vi "compile_options.vi"(8 "error in (no error)":errorcluster, 11 "Wash Options":T2) -> (0 "error out":errorcluster, 3 "Options Array":T1[](array[typedef]))   [LabVIEW 2021]
doc: "compile wash options into array"
uses:
  Controls/Wash Options.ctl
  Controls/states.ctl
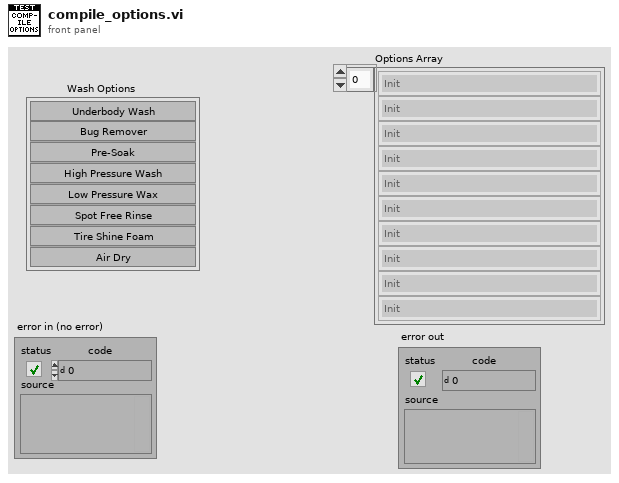
[diagram p1: front panel]
types:
  T1 = typedef "states.ctl" = enum16{"Init", "Select Wash Options", "Configure Options", "Under Body Wash", "Bug Remover", "Pre-Soak", "High Pressure Wash", "Low Pressure Wax", "Spot Free Rinse", "Tire Shine Foam", "Air Dry", "Skip", "Exit", "Stop"}
  T2 = typedef "Wash Options.ctl" = cluster{"Underbody Wash":bool, "Bug Remover":bool, "Pre-Soak":bool, "High Pressure Wash":bool, "Low Pressure Wax":bool, "Spot Free Rinse":bool, "Tire Shine Foam":bool, "Air Dry":bool}
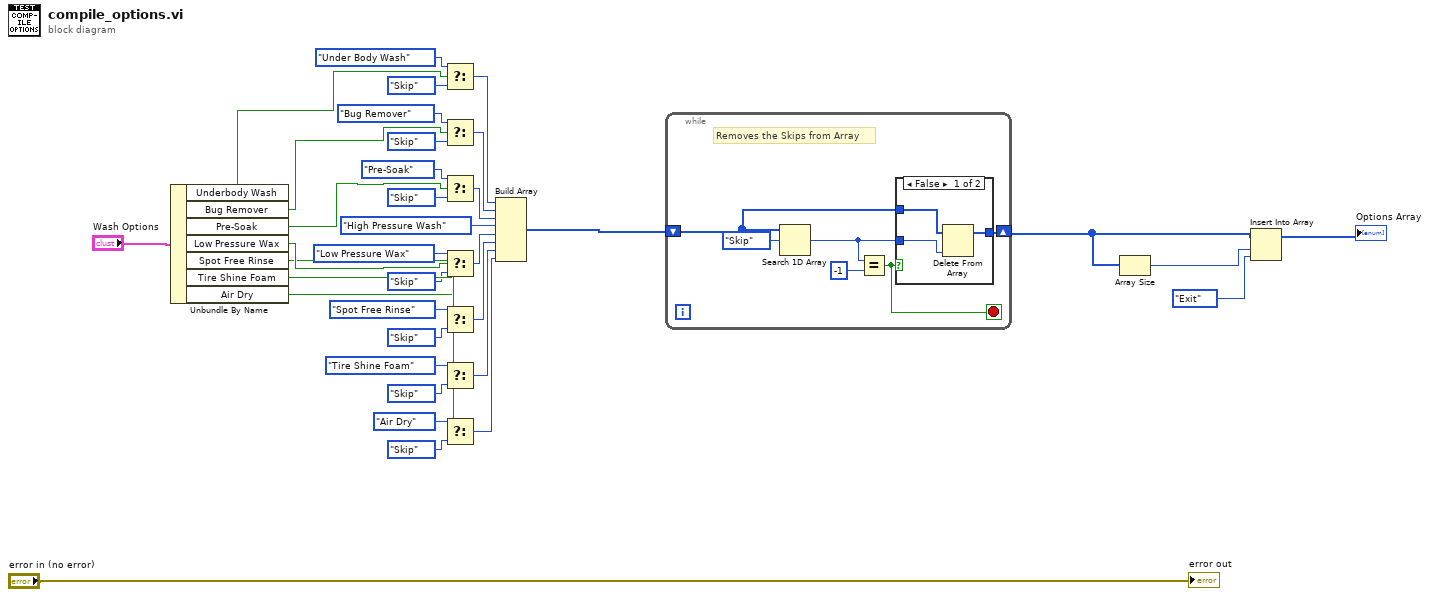
[diagram p0: block diagram]
diagram:
  n1 = Unbundle By Name("Wash Options") -> ("Underbody Wash"=w34:bool, "Bug Remover"=w27:bool, "Pre-Soak"=w26:bool, "Low Pressure Wax"=w25:bool, "Spot Free Rinse"=w24:bool, "Tire Shine Foam"=w23:bool, "Air Dry"=w22:bool)
  n2 = Select(t=states."Under Body Wash" ("Enum"), s=w34, f=states."Skip" ("Enum")) -> (s? t:f=w21:T1)
  n3 = Select(t=states."Bug Remover" ("Enum"), s=w27, f=states."Skip" ("Enum")) -> (s? t:f=w20:T1)
  n4 = Select(t=states."Pre-Soak" ("Enum"), s=w26, f=states."Skip" ("Enum")) -> (s? t:f=w19:T1)
  n5 = Select(t=states."Low Pressure Wax" ("Enum"), s=w25, f=states."Skip" ("Enum")) -> (s? t:f=w17:T1)
  n6 = Select(t=states."Spot Free Rinse" ("Enum"), s=w24, f=states."Skip" ("Enum")) -> (s? t:f=w16:T1)
  n7 = Select(t=states."Tire Shine Foam" ("Enum"), s=w23, f=states."Skip" ("Enum")) -> (s? t:f=w15:T1)
  n8 = Select(t=states."Air Dry" ("Enum"), s=w22, f=states."Skip" ("Enum")) -> (s? t:f=w14:T1)
  n9 = Build Array(w21, w20, w19, states."High Pressure Wash" ("Enum"), w17, w16, w15, w14) -> (w5:T1[])
  n10 = while {
    shift-right: [w38] -> w3
    shift-left: w5 -> [w41]
    stop <- w37 stop-if-true
    # "Removes the Skips from Array"
    n11 = Search 1D Array(1D array=w41, element=states."Skip") -> (index of element=w39:i32)  [unwired: 1 in]
    n12 = Equal?(x=w39, y=-1) -> (x = y?=w37:bool)
    n13 = case shown="False" w37 {
      tunnel: w41 -> [w45 w46]
      tunnel: w39 -> [w44 _]
      tunnel: [w43 w46] -> w38
      frame False {
        n14 = Delete From Array(array=w45, index=w44) -> (array with subset deleted=w43:T1[])  [unwired: 1 in, 1 out]
      }
      frame True {
      }
    }
  }
  n15 = Array Size(array=w3) -> (size(s)=w2:i32)
  n16 = Insert Into Array(array=w3, index=w2, new element=states."Exit" ("Enum")) -> (→"Options Array":T1[])
  "error out" <- "error in (no error)"
